vi "GUI_TapeDrive2.vi"() -> ()   [LabVIEW 2020]
uses:
  Device Drivers/TapeDrive/Mode_TypDEf.ctl
  Shared/Device Driver/OnOffTypeDef.ctl
  Device Drivers/TapeDrive/Direction_TypDef.ctl
  Shared/GUI_Template/GUI_master/tcp new data cluster.ctl
panel:
  in  "MaxStepTries::1":dbl=2.0 caption="MaxStepTries" min=0.0 max=10.0
  in  "tape monitor::1":T1 caption="PontingAndVertical\nCorrection"
  out "error out":errorcluster
  in  "WaitBeforeScanStep::1":dbl=5.0 caption="Step Wait ms" min=0.0 max=5000.0
  in  "SimpleMinTapeMonMaxCheck::1":T1 caption="Check TapeMon"
  in  "NumberSubSteps::1":dbl=5.0 caption="# SubSteps" min=0.0 max=5000.0
  in  "MinTapeMonMax::1":dbl=5.0 caption="MinCounts" min=0.0 max=4094.0
  in  "StepVelocity::1":dbl=5.0 caption="Step Velocity" min=0.0 max=0.5
  in  "OptimizeTensionAfterStep::1":T1 caption="Opt Tension after step"
  in  "MotorDirection::1":T2 caption="Direction"
  in  "direction::1":T2 caption="MasterSlave"
  in  "GUIdevice 1":string="PLM-PL1-TapeDrive"
  in  "TapeMotor::1":T1 caption="Tape Motors"
  in  "max velocity::1":dbl=5.0 caption="Max Velocity\ni.e tension" min=0.001 max=2000.0
  in  "stepsize::1":dbl=2.0 caption="Step Size" min=1.0 max=1000.0
  in  "Step::1":bool caption="Move Tape"
  in  "Mode::1":T3 caption="Mode"
  in  "Test Cluster":T4
  in  "stop":bool
  # "Tape Drive"
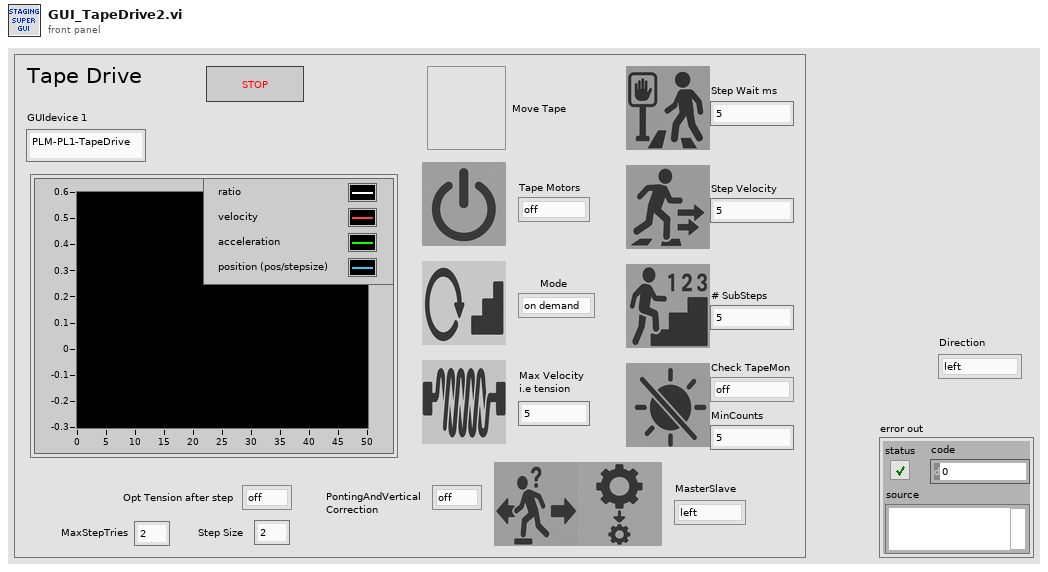
[diagram p1: front panel]
types:
  T1 = typedef "OnOffTypeDef.ctl" = enum16{"off", "on"}
  T2 = typedef "Direction_TypDef.ctl" = enum16{"left", "right"}
  T3 = typedef "Mode_TypDEf.ctl" = enum16{"on demand", "continuous", "scan"}
  T4 = cluster{"Channel::1":enum16{"Channel 0", "Channel 1", "Channel 2", "Channel 3"}, "Trajectory::1":waveform(dbl)[]}
  T5 = enum32{"invalid app kind", "Development System", "Run Time System", "Student Edition", "Embedded LabVIEW", "Evaluation", "Custom"}
  T6 = typedef "tcp new data cluster.ctl" = cluster{"EventEnum":enum16{"new data", "connection status update"}, "Device name":string}
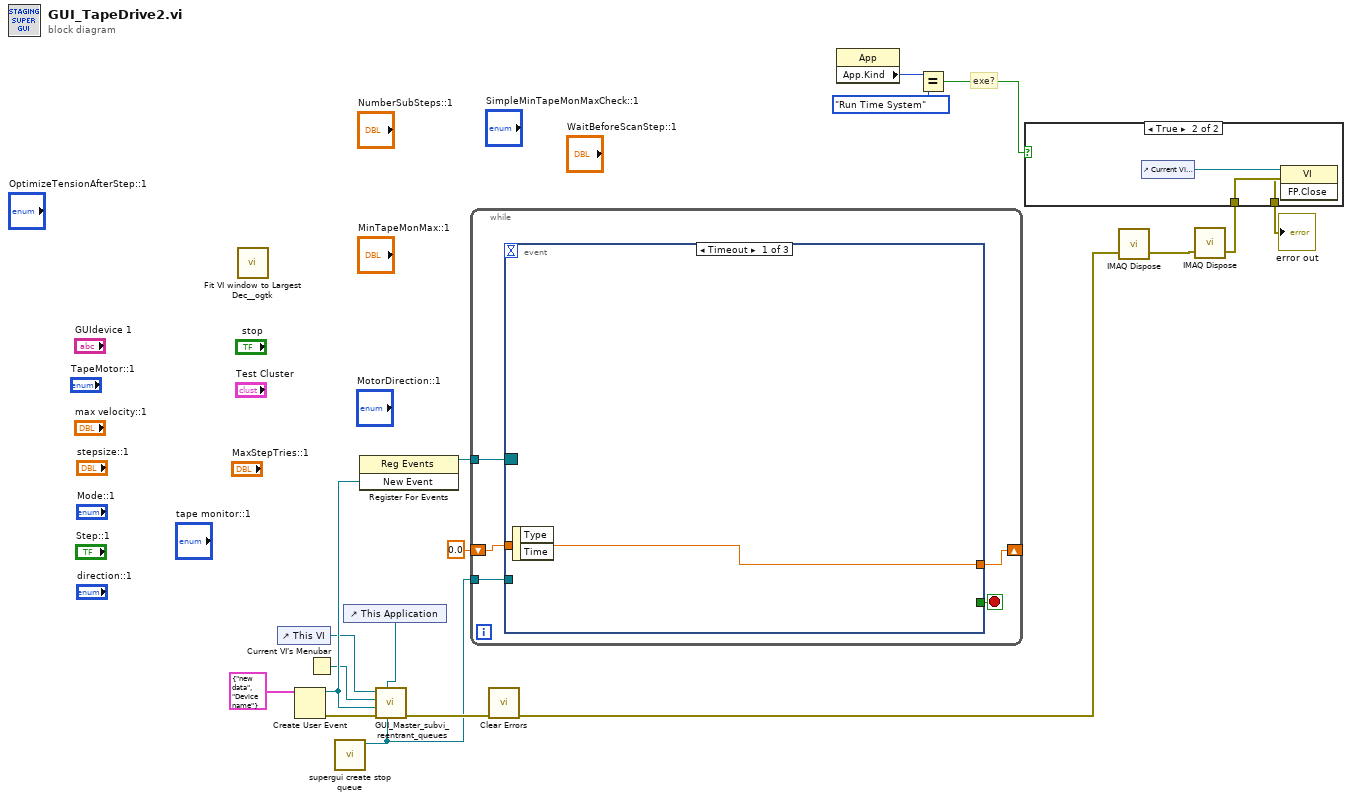
[diagram p0: block diagram]
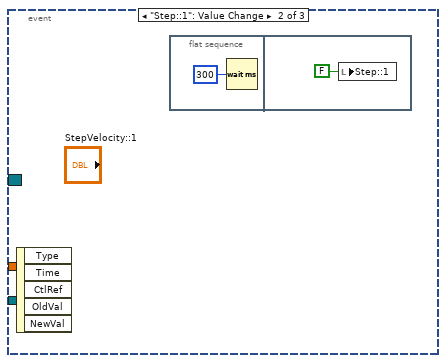
[diagram p3: hidden frame]
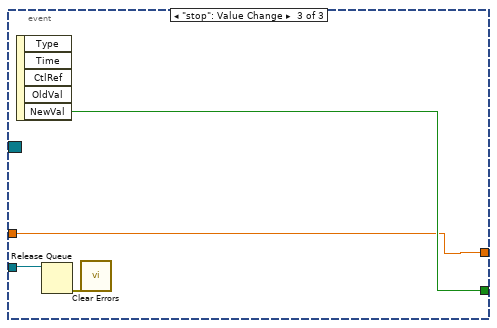
[diagram p4: hidden frame]
diagram:
  # "exe?"
  n1 = call <userlib>:"Fit VI window to Largest Dec__ogtk.vi"() -> ()  [unwired: 6 in, 2 out]
  n2 = control-ref of="This VI"() -> (w9:refnum<vi>)
  n3 = Create User Event(user event datatype=T6 {"EventEnum"=enum."new data", "Device name"="Device name"} ("New Event")) -> (user event=w14:refnum<user-event>, error out=w16:errorcluster)  [unwired: 1 in]
  n4 = Current VI's Menubar() -> (w8:refnum<k9>)
  n5 = call "supergui create stop queue.vi"() -> ("STOP Queue out"=w6:refnum<queue>)  [unwired: 11 in]
  n6 = control-ref of="This Application"() -> (w7:refnum<vi>)
  n7 = register-events(w14) -> (reference out=w13:refnum<event-registration>)  [unwired: 2 in, 1 out]
  n8 = call "GUI_Master_subvi_reentrant_queues.vi"("STOP Queue in"=w6, "This Application"=w7, "error in (no error)"=w16, "tcp data event"=w14, "Caller menu reference"=w8, "Caller VI ref"=w9) -> ("error out"=w15:errorcluster)  [unwired: 5 in]
  n9 = while {
    tunnel: w13 -> [w22]
    shift-right: [w19] -> _
    shift-left: 0.0 -> [w20]
    tunnel: w6 -> [w18]
    stop <- w21 stop-if-true
    n10 = event shown="[0] Timeout" {
      selector: w22 -> [_ _ _]
      dyn-events: _ -> [_ _ _]
      timeout: _ -> [_ _ _]
      tunnel: [_ _ w29] -> w21
      tunnel: w20 -> [w23 _ w28]
      tunnel: [w23 _ w28] -> w19
      tunnel: w18 -> [_ _ w27]
      event Timeout {
        n11 = event-data() -> ()  [unwired: 1 in, 2 out]
      }
      event "Step::1": Value Change {
        n12 = event-data() -> ()  [unwired: 1 in, 5 out]
        n13 = flat-sequence {
          frame #0 {
            n14 = Wait (ms)(milliseconds to wait=u32 300) -> ()  [unwired: 1 out]
          }
          frame #1 {
            n15 = local write "Step::1"(FALSE ("Step::1")) -> ()
          }
        }
      }
      event "stop": Value Change {
        n16 = event-data() -> ("NewVal"=w29:bool)  [unwired: 1 in, 4 out]
        n17 = Release Queue(queue=w27) -> (error out=w26:errorcluster)  [unwired: 2 in, 2 out]
        n18 = call <vilib>:"Clear Errors.vi"("error in (no error)"=w26) -> ()  [unwired: 5 in, 2 out]
      }
    }
  }
  n19 = call <vilib>:"Clear Errors.vi"("error in (no error)"=w15) -> ("error out"=w11:errorcluster)  [unwired: 5 in, 1 out]
  n20 = property class="App"() -> ("App.Kind"=w4:T5)  [unwired: 2 in, 2 out]
  n21 = Equal?(x=w4, y=T5."Run Time System" ("Application:Kind")) -> (x = y?=w2:bool)
  n22 = call "IMAQ Dispose"("error in (no error)"=w11) -> ("error out"=w10:errorcluster)  [unwired: 5 in]
  n23 = call "IMAQ Dispose"("error in (no error)"=w10) -> ("error out"=w5:errorcluster)  [unwired: 5 in]
  n24 = case shown="True" w2 {
    tunnel: w5 -> [w30 w33]
    tunnel: [w30 w31] -> w1
    frame False {
    }
    frame True {
      n25 = control-ref of="Current VI Reference"() -> (w32:refnum<vi>)
      n26 = invoke class="VI" method="FP.Close"(reference=w32, error in=w33) -> (error out=w31:errorcluster)  [unwired: 1 in, 2 out]
    }
  }
  "error out" <- w1
